vi "MKS_PDR2000_read_pressure.vi"(8 "error in (no error)":errorcluster, 11 "PDR2000 COM port":refnum<visa-resource-name>) -> (0 "error out":errorcluster, 3 "PDR2000 COM port out":refnum<visa-resource-name>, 4 "Channel 2 Pressure":dbl, 6 "Channel 1 Pressure":dbl)   [LabVIEW 2019]
uses:
  <vilib>/regexp/Match Regular Expression.xnode
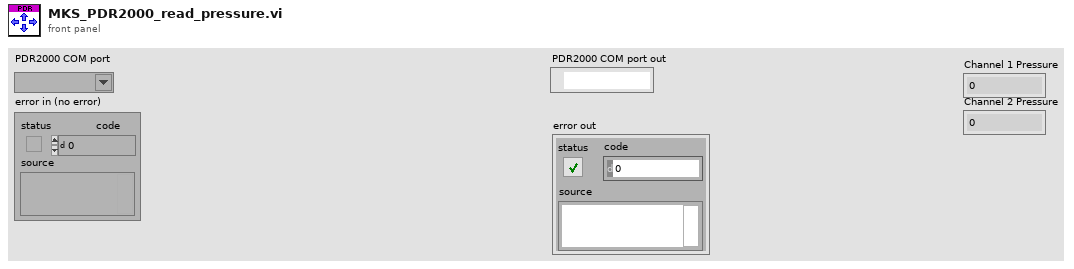
[diagram p1: front panel]
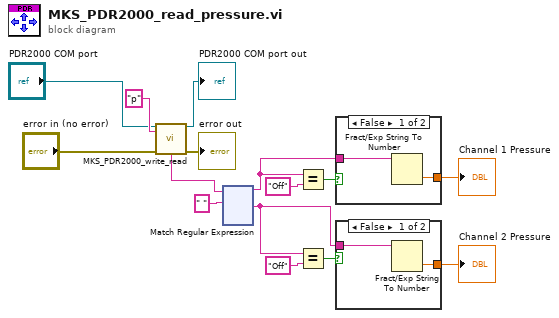
[diagram p0: block diagram]
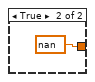
[diagram p2: hidden frame]
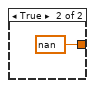
[diagram p3: hidden frame]
diagram:
  n1 = call "MKS_PDR2000_write_read.vi"("PDR2000 COM port"="PDR2000 COM port", "Write string"="p", "error in (no error)"="error in (no error)") -> ("PDR2000 COM port out"=→"PDR2000 COM port out":refnum<visa-resource-name>, "Read String"=w12:string, "error out"=→"error out":errorcluster)  [unwired: 10 in]
  n2 = xnode "Match Regular Expression"("input string"=w12, "regular expression"=" ") -> ("before match"=w1:string, "after match"=w8:string)  [unwired: 4 in, 3 out]
  n3 = Equal?(x=w1, y="Off") -> (x = y?=w4:bool)
  n4 = Equal?(x=w8, y="Off") -> (x = y?=w10:bool)
  n5 = case shown="False" w4 {
    tunnel: w1 -> [w17 _]
    tunnel: [w16 nan] -> w2
    frame False {
      n6 = Fract/Exp String To Number(string=w17) -> (number=w16:dbl)  [unwired: 3 in, 1 out]
    }
    frame True {
    }
  }
  "Channel 1 Pressure" <- w2
  n7 = case shown="False" w10 {
    tunnel: w8 -> [w20 _]
    tunnel: [w19 nan] -> w7
    frame False {
      n8 = Fract/Exp String To Number(string=w20) -> (number=w19:dbl)  [unwired: 3 in, 1 out]
    }
    frame True {
    }
  }
  "Channel 2 Pressure" <- w7
